vi "Save_plot_data (SubVI).vi"(6 "Save data":bool, 9 "String":string, 10 "Array":dbl[][](array[numeric]), 11 "File_name":path) -> ()   [LabVIEW 2020]
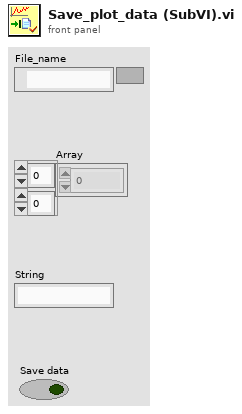
[diagram p1: front panel]
types:
  T1 = enum16{"open", "replace", "create", "open or create", "replace or create", "replace or create with confirmation"}
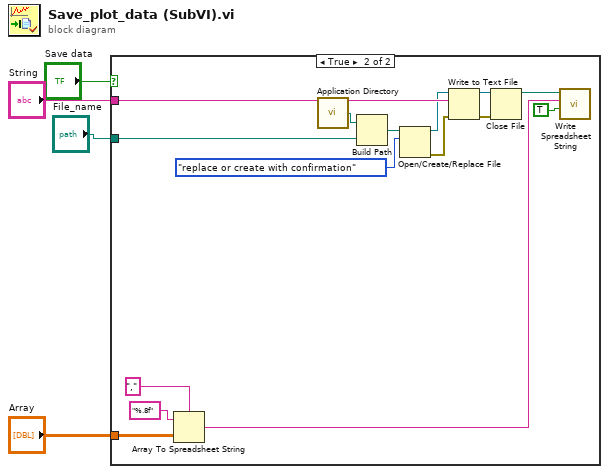
[diagram p0: block diagram]
diagram:
  n1 = case shown="True" "Save data" {
    tunnel: "Array" -> [_ w11]
    tunnel: "String" -> [_ w10]
    tunnel: "File_name" -> [_ w5]
    frame False {
    }
    frame True {
      n2 = Array To Spreadsheet String(delimiter (Tab)=",", array=w11, 3:"%.8f" ("format string")) -> (spreadsheet string=w18:string)
      n3 = call <vilib>:"Application Directory.vi"() -> ("Application Directory"=w16:path)
      n4 = Build Path(base path=w16, name or relative path=w5) -> (appended path=w15:path)
      n5 = Open/Create/Replace File(file path (use dialog)=w15, operation (0:open)=T1."replace or create with confirmation") -> (refnum out=w9:refnum<file>, error out=w8:errorcluster)  [unwired: 4 in, 1 out]
      n6 = Write to Text File(file (use dialog)=w9, text=w10, error in=w8) -> (refnum out=w7:refnum<file>, error out=w6:errorcluster)  [unwired: 1 in, 1 out]
      n7 = Close File(refnum=w7, error in=w6) -> (path=w14:path)  [unwired: 1 out]
      n8 = call <vilib>:"Write Spreadsheet String.vi"("append to file? (new file:F)"=TRUE, "spreadsheet string"=w18, "file path (dialog if empty)"=w14) -> ()  [unwired: 7 in, 2 out]
    }
  }
